vi "Set Step.vi"(7 "Processing Step":T1, 10 "RequestTraceLog in":refnum<class "RequestTraceLog.lvclass">) -> (2 "RequestTraceLog out":refnum<class "RequestTraceLog.lvclass">)   [LabVIEW 2020, in "HTTP Server.lvlib" / "RequestTraceLog.lvclass"]
uses:
  RequestTraceLog.lvclass
  Processing Step.ctl
  HTTP Server.lvlib
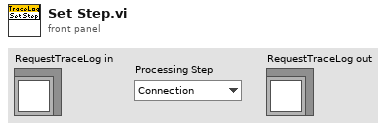
[diagram p1: front panel]
types:
  T1 = typedef "HTTP Server.lvlib/Processing Step.ctl" = enum16{"Connection", "Request", "Routing", "Controller Init", "Controller", "Response", "Complete", "Exception"}
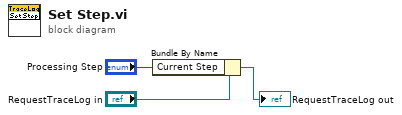
[diagram p0: block diagram]
diagram:
  n1 = Bundle By Name(cluster="RequestTraceLog in", "Current Step"="Processing Step") -> (→"RequestTraceLog out":refnum<class "RequestTraceLog.lvclass">)
